vi "Config data to Writable Controls.vi"(8 "error in (no error)":errorcluster, 10 "Config Data":T1={"DS First Launch"=FALSE, "LogBaseFolder"=path "", "Live Logging"=FALSE, "Server Port"=0, "Max Number ML Rows"=0, "AM.WinBounds"={"Left"=0, "Top"=0, "Right"=0, "Bottom"=0}, "AM.FP.State"=enum."Invalid", "AM.Monitor"=0, "AM.Column Widths"=[], "ML.Visible Columns"=[], "ML.Splitter Position"=0, "ML.Column Widths"=[], "ML.WinBounds"={"Left"=0, "Top"=0, "Right"=0, "Bottom"=0}, "ML.FP.State"=enum."Invalid", "ML.Monitor"=0}, 11 "Settings in":refnum<class "Settings.lvclass">) -> (0 "error out":errorcluster, 3 "Settings out":refnum<class "Settings.lvclass">)   [LabVIEW 2017, in "Settings.lvclass"]
uses:
  Settings.lvclass
  Config Data.ctl
  <vilib>/Utility/miscctls.llb/LVRectTypeDef.ctl
  Settings.lvclass/Settings.ctl
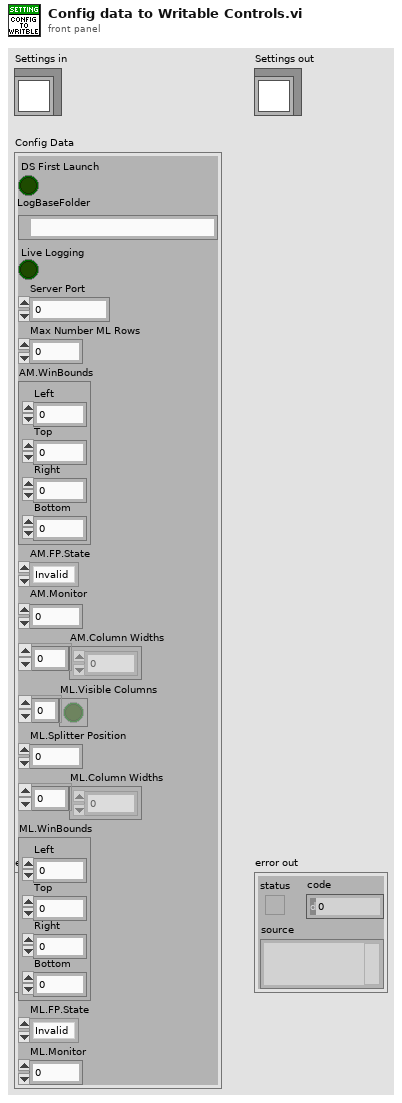
[diagram p1: front panel]
types:
  T1 = typedef "Settings.lvclass/Config Data.ctl" = cluster{"DS First Launch":bool, "LogBaseFolder":path, "Live Logging":bool, "Server Port":u16, "Max Number ML Rows":i32, "AM.WinBounds":T2, "AM.FP.State":enum32{"Invalid", "Standard", "Closed", "Hidden", "Minimized", "Maximized"}, "AM.Monitor":u16, "AM.Column Widths":u32[], "ML.Visible Columns":bool[], "ML.Splitter Position":i32, "ML.Column Widths":u32[], "ML.WinBounds":T2, "ML.FP.State":enum32{"Invalid", "Standard", "Closed", "Hidden", "Minimized", "Maximized"}, "ML.Monitor":u16}
  T2 = typedef "LVRectTypeDef.ctl" = cluster{"Left":i16, "Top":i16, "Right":i16, "Bottom":i16}
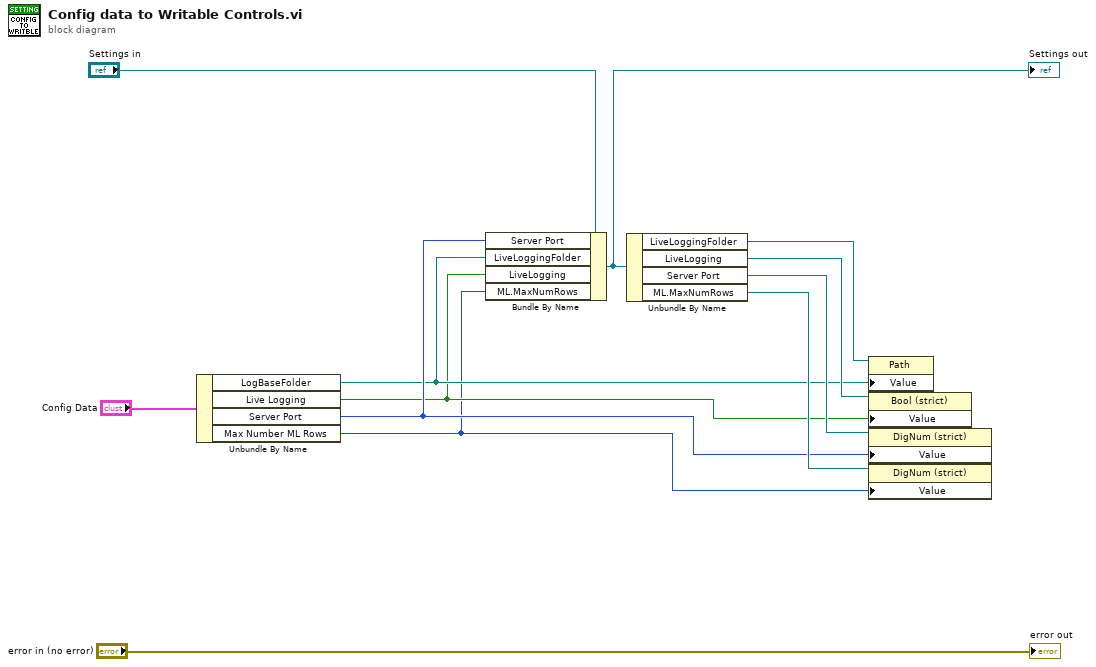
[diagram p0: block diagram]
diagram:
  n1 = Unbundle By Name("Config Data") -> ("LogBaseFolder"=w3:path, "Live Logging"=w2:bool, "Server Port"=w4:u16, "Max Number ML Rows"=w1:i32)
  n2 = Bundle By Name(cluster="Settings in", "Server Port"=w4, "LiveLoggingFolder"=w3, "LiveLogging"=w2, "ML.MaxNumRows"=w1) -> (w5:refnum<class "Settings.lvclass">)
  "Settings out" <- w5
  n3 = Unbundle By Name(w5) -> ("LiveLoggingFolder"=w8:refnum<vi>, "LiveLogging"=w7:refnum<vi>, "Server Port"=w9:refnum<vi>, "ML.MaxNumRows"=w6:refnum<vi>)
  n4 = property class="Path"(reference=w8, "Value"=w3) -> ()  [unwired: 1 in, 2 out]
  n5 = property class="Bool (strict)"(reference=w7, "Value"=w2) -> ()  [unwired: 1 in, 2 out]
  n6 = property class="DigNum (strict)"(reference=w9, "Value"=w4) -> ()  [unwired: 1 in, 2 out]
  n7 = property class="DigNum (strict)"(reference=w6, "Value"=w1) -> ()  [unwired: 1 in, 2 out]
  "error out" <- "error in (no error)"
